vi "Initialize.vi"(8 "error in":errorcluster, 9 "parameters":variant, 10 "path":path, 11 "repository in":refnum<class "modification container.lvclass">) -> (0 "error out":errorcluster, 3 "repository out":refnum<class "modification container.lvclass">)   [LabVIEW 2013, in "modification container.lvclass"]
doc: "Initializes the repo. StoreClassPath method should be called in this VI"
uses:
  modification container.lvclass
  <vilib>/CEF_TreeControl/Repository/NISE_CEF_Repository.lvclass
  VI modification.lvclass
  collection/available modifications.vi
  collection/VI modification collection.lvclass
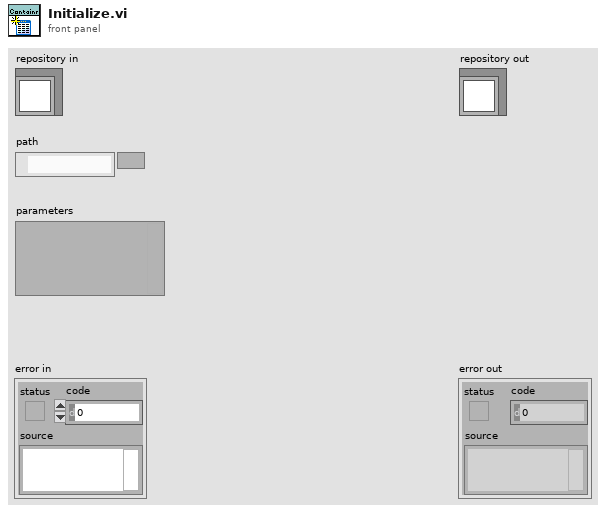
[diagram p1: front panel]
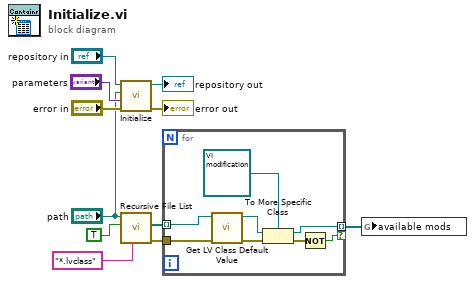
[diagram p0: block diagram]
diagram:
  n1 = call-parent "Initialize.vi"("error in"="error in", "parameters"="parameters", "path"="path", "repository in"="repository in") -> ("error out"=→"error out":errorcluster, "repository out"=→"repository out":refnum<class "modification container.lvclass">)  [unwired: 6 in]
  n2 = call <vilib>:"Recursive File List.vi"("pattern"="*.lvclass", "Treat LLBs as Folders?"=TRUE, "Folder Path"="path") -> ("error out"=w2:errorcluster, "All Files in Dir"=w1:path[])  [unwired: 4 in, 3 out]
  n3 = for {
    tunnel: [w18] -> w3 mode=indexing if=w16
    tunnel: w2 -> [w15]
    tunnel: w1 -> [w14] mode=indexing
    n4 = call <vilib>:"Get LV Class Default Value.vi"("error in (no error)"=w15, "class path"=w14) -> ("error out"=w12:errorcluster, "object"=w13:refnum<class>)  [unwired: 8 in]
    n5 = To More Specific Class(target class=refnum<class "VI modification.lvclass"> refnum ("VI modification"), reference=w13, error in=w12) -> (specific class reference=w18:refnum<class "VI modification.lvclass">, error out=w17:errorcluster)
    n6 = Not(x=w17) -> (.not. x?=w16:bool)
  }
  n7 = global write "available modifications.vi" "available mods"(w3) -> ()
